vi "Write and Read Digital Output.vi"(8 "error in (no error)":errorcluster, 10 "initial channel settings":T1[](array[typedef]), 11 "Scan Engine Scripting API Modules in":refnum<class "Scan Engine Scripting API Modules.lvclass">) -> (0 "error out":errorcluster, 2 "read channel settings":T1[](array[typedef]), 3 "Scan Engine Scripting API Modules out":refnum<class "Scan Engine Scripting API Modules.lvclass">)   [LabVIEW 2020, in "Scan Engine Scripting API Modules.lvclass"]
uses:
  Scan Engine Scripting API Modules.lvclass
  Scripting/Modules/Mode Classes/Controls/digital channel settings.ctl
  Scripting/Scan Engine Scripting.lvlib
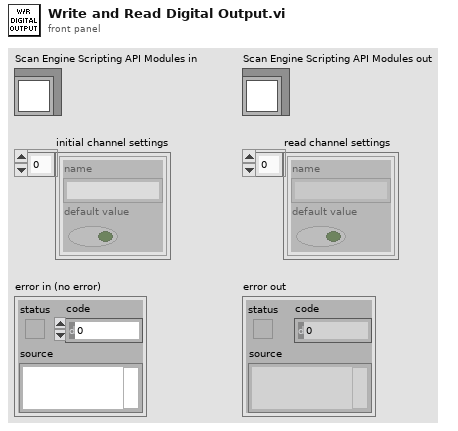
[diagram p1: front panel]
types:
  T1 = typedef "Scan Engine Scripting.lvlib/digital channel settings.ctl" = cluster{"name":string, "default value":bool}
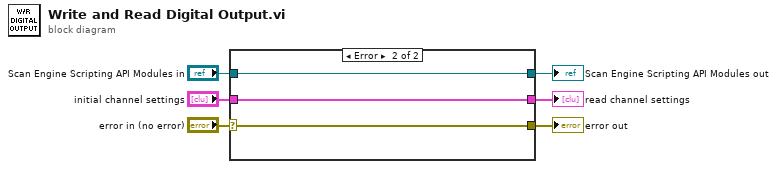
[diagram p0: block diagram]
diagram:
  n1 = case shown="Error" "error in (no error)" {
    selector: "error in (no error)" -> [w8 w12]
    tunnel: [w8 w12] -> w5
    tunnel: [w9 w11] -> w3
    tunnel: "Scan Engine Scripting API Modules in" -> [w9 w11]
    tunnel: "initial channel settings" -> [w7 w10]
    tunnel: [w7 w10] -> w1
    frame No Error {
      # "Wire the error cluster across even in the \"No Error\"\ncase so that warnings get propagated."
    }
    frame Error {
    }
  }
  "error out" <- w5
  "Scan Engine Scripting API Modules out" <- w3
  "read channel settings" <- w1
